vi "Acquisition Message Loop.vi"(8 "error in (no error)":errorcluster, 9 "Data Queue":refnum<queue>, 10 "Data Notifier":refnum<notifier>, 11 "Message Queues":T1) -> (0 "error out":errorcluster)   [LabVIEW 2014, in "PLS Acquisition.lvlib"]
doc: "Message loop for handling messages pertaining to the acquisition of data from the hardware."
uses:
  PLS Acquisition.lvlib
  support/Message Queue/All Message Queues.ctl
  support/Message Queue/Message Cluster.ctl
  Hardware Configuration.ctl
  Settings/conversion.ctl
  Acquisition State.ctl
  <vilib>/DAQmx/write.llb/DAQmx Write (Digital 1D Bool NChan 1Samp 1Line).vi
  support/Message Queue/Enqueue Message (Single).vi
  <vilib>/DAQmx/miscellaneous.llb/DAQmx Fill In Error Info.vi
  <vilib>/Utility/error.llb/Error Cluster From Error Code.vi
  <vilib>/ErrorRing/Error Ring.xnode
  support/Message Queue/PLS Message Queue.lvlib
  Settings/PLS Settings.lvlib
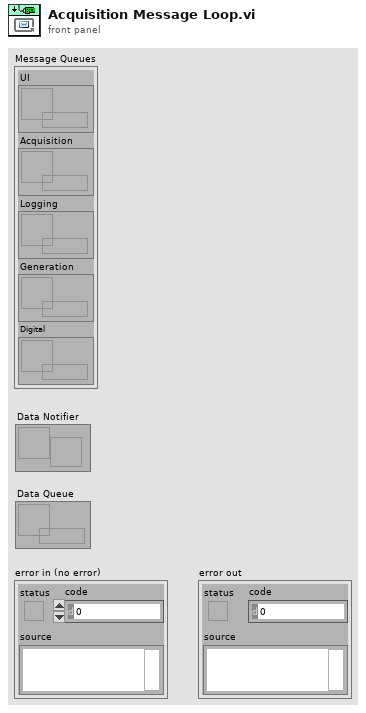
[diagram p1: front panel]
types:
  T1 = typedef "PLS Message Queue.lvlib/All Message Queues.ctl" = cluster{"UI":refnum<queue>, "Acquisition":refnum<queue>, "Logging":refnum<queue>, "Generation":refnum<queue>, "Digital":refnum<queue>}
  T2 = typedef "PLS Acquisition.lvlib/Hardware Configuration.ctl" = cluster{"AI":cluster{"task name":string, "task_ref":refnum<k21>, "physical channels":tag, "channels config":cluster{"input terminal configuration":i32, "minimum value":dbl, "maximum value":dbl}, "rate":dbl}, "conversions":cluster{"ai0":T3, "ai1":T3, "ai2":T3, "ai3":T3, "ai4":T3}, "compteur 0":cluster{"task name":string, "task_ref":refnum<k21>, "ctr":tag, "coeff":dbl}, "compteur 1":cluster{"task name":string, "task_ref":refnum<k21>, "ctr":tag, "coeff":dbl}, "compteur 2":cluster{"task name":string, "task_ref":refnum<k21>, "ctr":tag, "coeff":dbl}, "compteur 3":cluster{"task name":string, "task_ref":refnum<k21>, "ctr":tag, "coeff":dbl}}
  T3 = typedef "PLS Settings.lvlib/conversion.ctl" = cluster{"a":dbl, "b":dbl}
  T4 = typedef "PLS Acquisition.lvlib/Acquisition State.ctl" = enum16{"Idle", "Acquiring"}
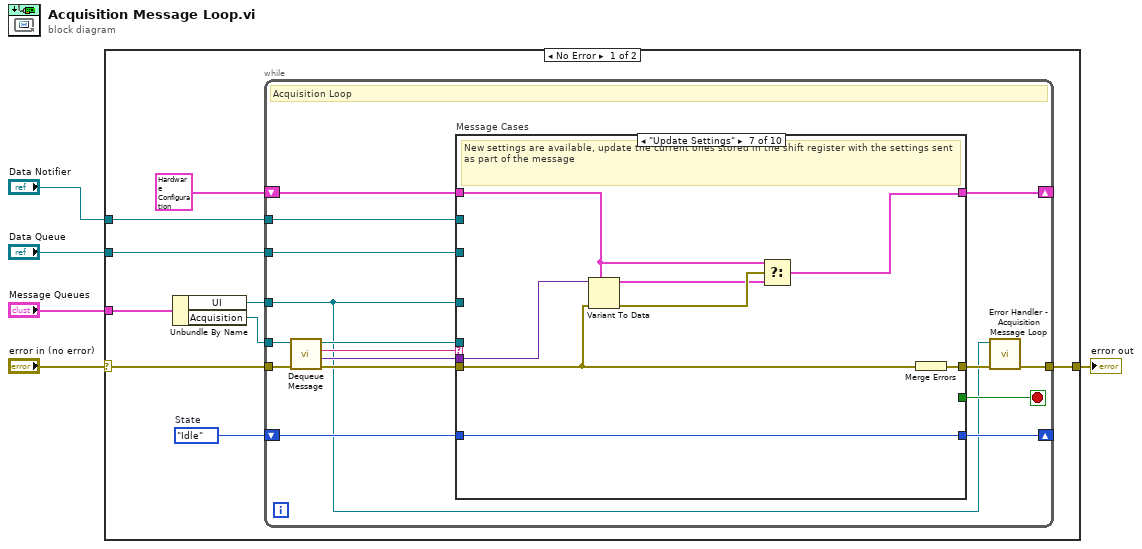
[diagram p0: block diagram]
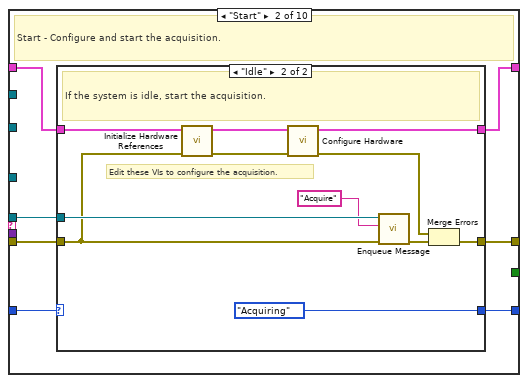
[diagram p3: hidden frame]
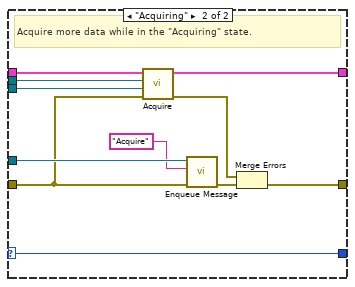
[diagram p6: hidden frame]
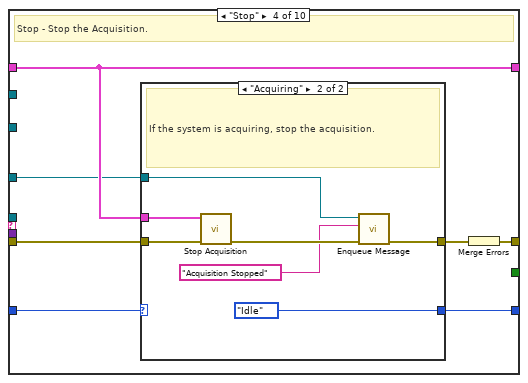
[diagram p7: hidden frame]
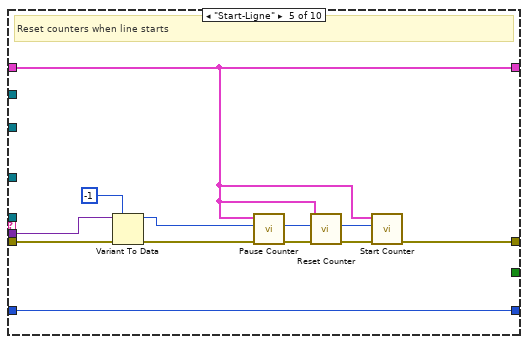
[diagram p9: hidden frame]
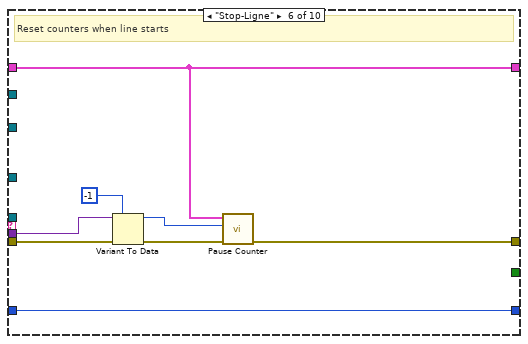
[diagram p10: hidden frame]
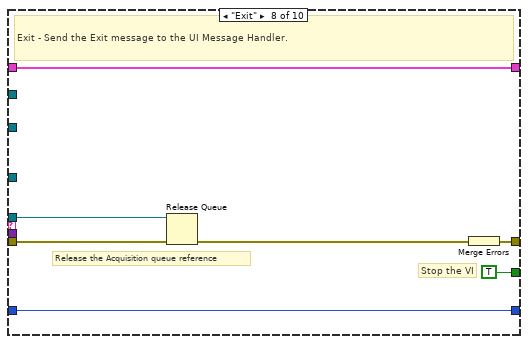
[diagram p11: hidden frame]
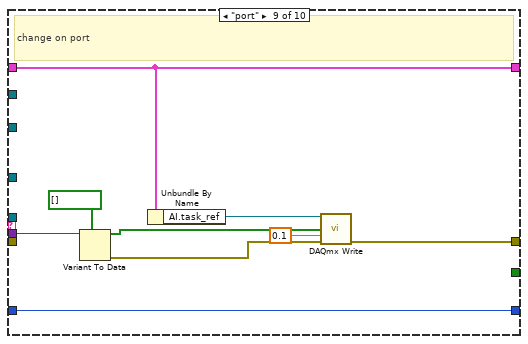
[diagram p12: hidden frame]
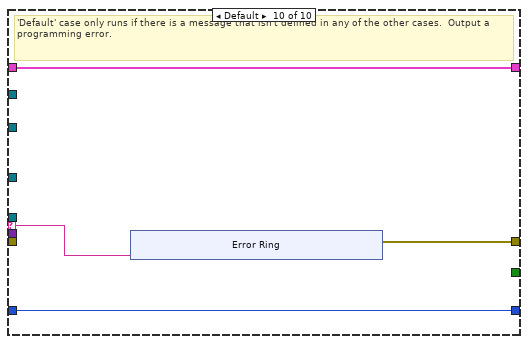
[diagram p13: hidden frame]
diagram:
  n1 = case shown="No Error" "error in (no error)" {
    selector: "error in (no error)" -> [w10 w147]
    tunnel: "Message Queues" -> [w14 _]
    tunnel: [w12 w147] -> w4
    tunnel: "Data Notifier" -> [w8 _]
    tunnel: "Data Queue" -> [w7 _]
    frame No Error {
      w6 = Acquisition_State."Idle"  # State
      n2 = Unbundle By Name(w14) -> ("UI"=w9:refnum<queue>, "Acquisition"=w13:refnum<queue>)
      n3 = while {
        tunnel: w13 -> [w23]
        shift-right: [w29] -> _
        shift-left: T2 {"AI"={"task name"="AI", "task_ref"="", "physical channels"="Dev1/ai0:4", "channels config"={"input terminal configuration"=10083, "minimum value"=-5.0, "maximum value"=5.0}, "rate"=1000.0}, "conversions"={"ai0"={"a"=1.0, "b"=0.0}, "ai1"={"a"=1.0, "b"=0.0}, "ai2"={"a"=1.0, "b"=0.0}, "ai3"={"a"=1.0, "b"=0.0}, "ai4"={"a"=1.0, "b"=0.0}}, "compteur 0"={"task name"="CTR", "task_ref"="", "ctr"="Dev1/ctr0:3", "coeff"=4000.0}, "compteur 1"={"task name"="CTR1", "task_ref"="", "ctr"="Dev1/ctr1", "coeff"=4000.0}, "compteur 2"={"task name"="CTR2", "task_ref"="", "ctr"="Dev1/ctr2", "coeff"=4000.0}, "compteur 3"={"task name"="CTR3", "task_ref"="", "ctr"="Dev1/ctr3", "coeff"=4000.0}} ("Data Cluster") -> [w30]
        tunnel: w9 -> [w15]
        tunnel: w8 -> [w22]
        tunnel: w7 -> [w21]
        shift-right: [w19] -> _
        shift-left: w6 -> [w20]
        tunnel: w10 -> [w27]
        tunnel: [w18] -> w12
        stop <- w28 stop-if-true
        # "Acquisition Loop"
        n4 = call "Dequeue Message.vi"("error in (no error)"=w27, "Message Queue"=w23) -> ("error out"=w26:errorcluster, "Message Data"=w24:variant, "Message"=w25:string, "dup Message Queue"=w16:refnum<queue>)  [unwired: 6 in]
        n5 = case "Message Cases" shown="\"Update Settings\"" w25 {
          selector: w25 -> [_ _ _ _ _ _ _ _ _ w136]
          tunnel: w16 -> [_ w37 w62 _ _ _ _ w121 _ _]
          tunnel: w26 -> [w32 w38 w61 w83 w102 w108 w115 w123 _ _]
          tunnel: [w32 w40 w63 w84 w98 w109 w119 w125 w128 w137] -> w17
          tunnel: w30 -> [w31 w39 w59 w81 w95 w110 w113 w124 w134 w139]
          tunnel: [w31 w36 w60 w81 w95 w110 w112 w124 w134 w139] -> w29
          tunnel: [_ _ _ _ _ _ _ TRUE _ _] -> w28
          tunnel: w24 -> [_ _ _ _ w100 w105 w118 _ w133 _]
          tunnel: w15 -> [_ _ _ w78 _ _ _ _ _ _]
          tunnel: w22 -> [_ _ w58 _ _ _ _ _ _ _]
          tunnel: w21 -> [_ _ w57 _ _ _ _ _ _ _]
          tunnel: w20 -> [w33 w34 w55 w80 w103 w111 w114 w120 w135 w138]
          tunnel: [w33 w35 w56 w79 w103 w111 w114 w120 w135 w138] -> w19
          frame "Initialize" {
            # "Initialize  - Initialize is currently a no-op.  The hardware initialization takes place in the 'Start' message."
          }
          frame "Start" {
            # "Start - Configure and start the acquisition."
            n6 = case shown="\"Idle\"" w34 {
              selector: w34 -> [w41 _]
              tunnel: [w42 w54] -> w40
              tunnel: w39 -> [w43 w47]
              tunnel: w38 -> [w42 w46]
              tunnel: w37 -> [_ w52]
              tunnel: [w43 w50] -> w36
              tunnel: [w41 Acquisition_State."Acquiring" ("Acquisition State")] -> w35
              frame "Acquiring" {
                # "The system is already acquiring. Ignore the \"Start\" message."
              }
              frame "Idle" {
                # "Edit these VIs to configure the acquisition."
                # "If the system is idle, start the acquisition."
                n7 = call "Initialize Hardware References.vi"("error in (no error)"=w46, "Hardware Resources in"=w47) -> ("error out"=w45:errorcluster, "Hardware Resources out"=w44:T2)  [unwired: 8 in]
                n8 = call "Configure Hardware.vi"("error in (no error)"=w45, "Hardware Resources in"=w44) -> ("error out"=w51:errorcluster, "Hardware Resources out"=w50:T2)  [unwired: 8 in]
                n9 = call-poly "Enqueue Message.vi"("error in (no error)"=w46, "Message"="Acquire", "Message Queue"=w52) -> ("error out"=w53:errorcluster)  [unwired: 7 in, 1 out]
                n10 = Merge Errors(w51, w53) -> (w54:errorcluster)
              }
            }
          }
          frame "Acquire" {
            # "Acquire - Acquire data from the hardware. Since this is a continuous acquisition, this message will always message itself to run again."
            n11 = case shown="\"Idle\"" w55 {
              selector: w55 -> [w64 w68]
              tunnel: [w65 w77] -> w63
              tunnel: w62 -> [_ w75]
              tunnel: w61 -> [w65 w67]
              tunnel: [w66 w73] -> w60
              tunnel: w59 -> [w66 w72]
              tunnel: w58 -> [_ w70]
              tunnel: w57 -> [_ w69]
              tunnel: [w64 w68] -> w56
              frame "Idle" {
                # "Ignore \"Acquire\" messages when the acquisition is idle."
              }
              frame "Acquiring" {
                # "Acquire more data while in the \"Acquiring\" state."
                n12 = call "Acquire.vi"("error in (no error)"=w67, "Data Queue"=w69, "Data Notifier"=w70, "Hardware Resources in"=w72) -> ("error out"=w74:errorcluster, "Hardware Resources out"=w73:T2)  [unwired: 6 in]
                n13 = call-poly "Enqueue Message.vi"("error in (no error)"=w67, "Message"="Acquire", "Message Queue"=w75) -> ("error out"=w76:errorcluster)  [unwired: 7 in, 1 out]
                n14 = Merge Errors(w74, w76) -> (w77:errorcluster)
              }
            }
          }
          frame "Stop" {
            # "Stop - Stop the Acquisition."
            n15 = case shown="\"Acquiring\"" w80 {
              selector: w80 -> [w85 _]
              tunnel: w83 -> [w86 w93]
              tunnel: [w86 w89] -> w82
              tunnel: w81 -> [_ w91]
              tunnel: [w85 Acquisition_State."Idle" ("State")] -> w79
              tunnel: w78 -> [_ w88]
              frame "Idle" {
                # "The system is already idle. Ignore the \"Stop\" message."
              }
              frame "Acquiring" {
                # "If the system is acquiring, stop the acquisition."
                n16 = call "Stop Acquisition.vi"("error in (no error)"=w93, "Hardware Resources in"=w91) -> ("error out"=w92:errorcluster)  [unwired: 9 in]
                n17 = call-poly "Enqueue Message.vi"("error in (no error)"=w92, "Message"="Acquisition Stopped", "Message Queue"=w88) -> ("error out"=w89:errorcluster)  [unwired: 7 in, 1 out]
              }
            }
            n18 = Merge Errors(w82) -> (w84:errorcluster)
          }
          frame "Start-Ligne" {
            # "Reset counters when line starts"
            n19 = Variant To Data(error in=w102, type=-1 ("ligne index"), Variant=w100) -> (data=w96:i32, error out=w97:errorcluster)
            n20 = call "Pause Counter.vi"("error in (no error)"=w97, "ligne index"=w96, "Hardware Resources in"=w95) -> ("error out"=w94:errorcluster)  [unwired: 7 in, 1 out]
            n21 = call "Reset Counter.vi"("error in (no error)"=w94, "ligne index"=w96, "Hardware Resources in"=w95) -> ("error out"=w99:errorcluster)  [unwired: 8 in]
            n22 = call "Start Counter.vi"("error in (no error)"=w99, "ligne index"=w96, "Hardware Resources in"=w95) -> ("error out"=w98:errorcluster)  [unwired: 8 in]
          }
          frame "Stop-Ligne" {
            # "Reset counters when line starts"
            n23 = Variant To Data(error in=w108, type=-1 ("ligne index"), Variant=w105) -> (data=w104:i32, error out=w107:errorcluster)
            n24 = call "Pause Counter.vi"("error in (no error)"=w107, "ligne index"=w104, "Hardware Resources in"=w110) -> ("error out"=w109:errorcluster)  [unwired: 7 in, 1 out]
          }
          frame "Update Settings" {
            # "New settings are available, update the current ones stored in the shift register with the settings sent as part of the message"
            n25 = Variant To Data(error in=w115, type=w113, Variant=w118) -> (data=w116:T2, error out=w117:errorcluster)
            n26 = Select(t=w113, s=w117, f=w116) -> (s? t:f=w112:T2)
            n27 = Merge Errors(w115) -> (w119:errorcluster)
          }
          frame "Exit" {
            # "Release the Acquisition queue reference"
            # "Stop the VI"
            # "Exit - Send the Exit message to the UI Message Handler."
            n28 = Release Queue(queue=w121, error in (no error)=w123) -> (error out=w122:errorcluster)  [unwired: 1 in, 2 out]
            n29 = Merge Errors(w122) -> (w125:errorcluster)
          }
          frame "port" {
            # "change on port"
            n30 = Variant To Data(type=bool[] [], Variant=w133) -> (data=w131:bool[], error out=w129:errorcluster)  [unwired: 1 in]
            n31 = Unbundle By Name(w134) -> ("AI.task_ref"=w130:refnum<k21>)
            n32 = call-poly <vilib>:"DAQmx Write.vi"("task/channels in"=w130, "data"=w131, "timeout"=0.1, "error in"=w129) -> ("error out"=w128:errorcluster)  [unwired: 9 in, 2 out]
          }
          frame Default {
            # "'Default' case only runs if there is a message that isn't defined in any of the other cases.  Output a programming error."
            n33 = xnode "Error Ring"("parameter 0"=w136) -> ("error out"=w137:errorcluster)
          }
        }
        n34 = call "Error Handler - Acquisition Message Loop.vi"("error in (no error)"=w17, "Message Queue"=w15) -> ("dup error in"=w18:errorcluster)  [unwired: 8 in, 1 out]
      }
    }
    frame Error {
    }
  }
  "error out" <- w4
